vi "Data_PSD( Current Signal).vi"() -> ()   [LabVIEW 2020]
doc: "Use this template to build a producer/consumer design pattern. Use this template when you need to execute a process, such as data analysis, when a data source, such as a triggered acquisition, produces data at an uneven rate and you need to execute the process when the data becomes available."
uses:
  <vilib>/Utility/error.llb/DialogType.ctl
  <vilib>/measure/maspectr.llb/Power Spectrum and PSD Export Mode.ctl
  <vilib>/Analysis/4window.llb/windowTd.ctl
  <vilib>/DAQmx/read.llb/DAQmx Read (Analog Wfm 1Chan NSamp).vi
  <vilib>/DAQmx/create/channels.llb/DAQmx Create Channel (AI-Voltage-Basic).vi
  <vilib>/DAQmx/configure/timing.llb/DAQmx Timing (Sample Clock).vi
  <vilib>/DAQmx/miscellaneous.llb/DAQmx Fill In Error Info.vi
  <vilib>/measure/maspectr.llb/FFT Power Spectrum and PSD for 1 Chan.vi
  <vilib>/Analysis/0measdsp.llb/Scaled Time Domain Window (DBL).vi
  <vilib>/Analysis/NI_AALPro.lvlib
  <vilib>/measure/NI_MAPro.lvlib
panel:
  out "size(s)":i32
  out "Signal 2":waveform(dbl)(graph)
  in  "stop":bool
  out "Numeric":i32
  out "Signal":waveform(dbl)(graph)
  out "Max Amplitude":dbl
  out "PSD of Signal":cluster{"f0":dbl, "df":dbl, "S(f)":dbl[]}(graph)
  out "Frequency Peak":dbl format="%0.4f"
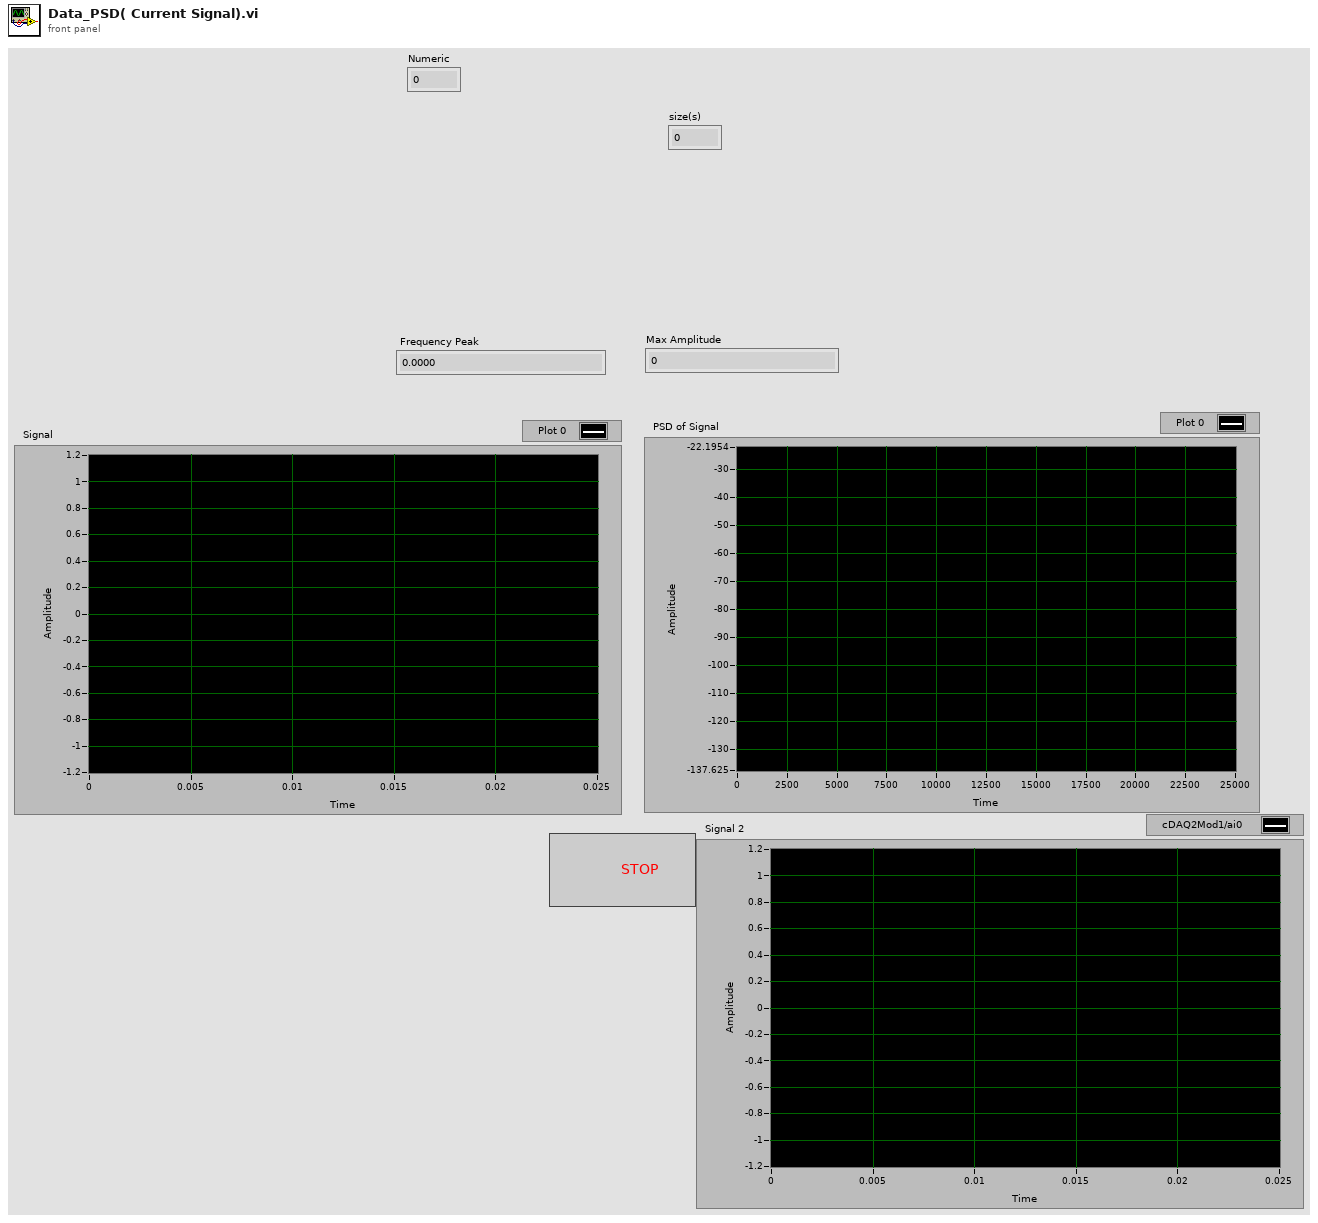
[diagram p1: front panel]
types:
  T1 = typedef "DialogType.ctl" = u16
  T2 = typedef "NI_AALPro.lvlib/windowTd.ctl" = u32
  T3 = typedef "NI_MAPro.lvlib/Power Spectrum and PSD Export Mode.ctl" = u16
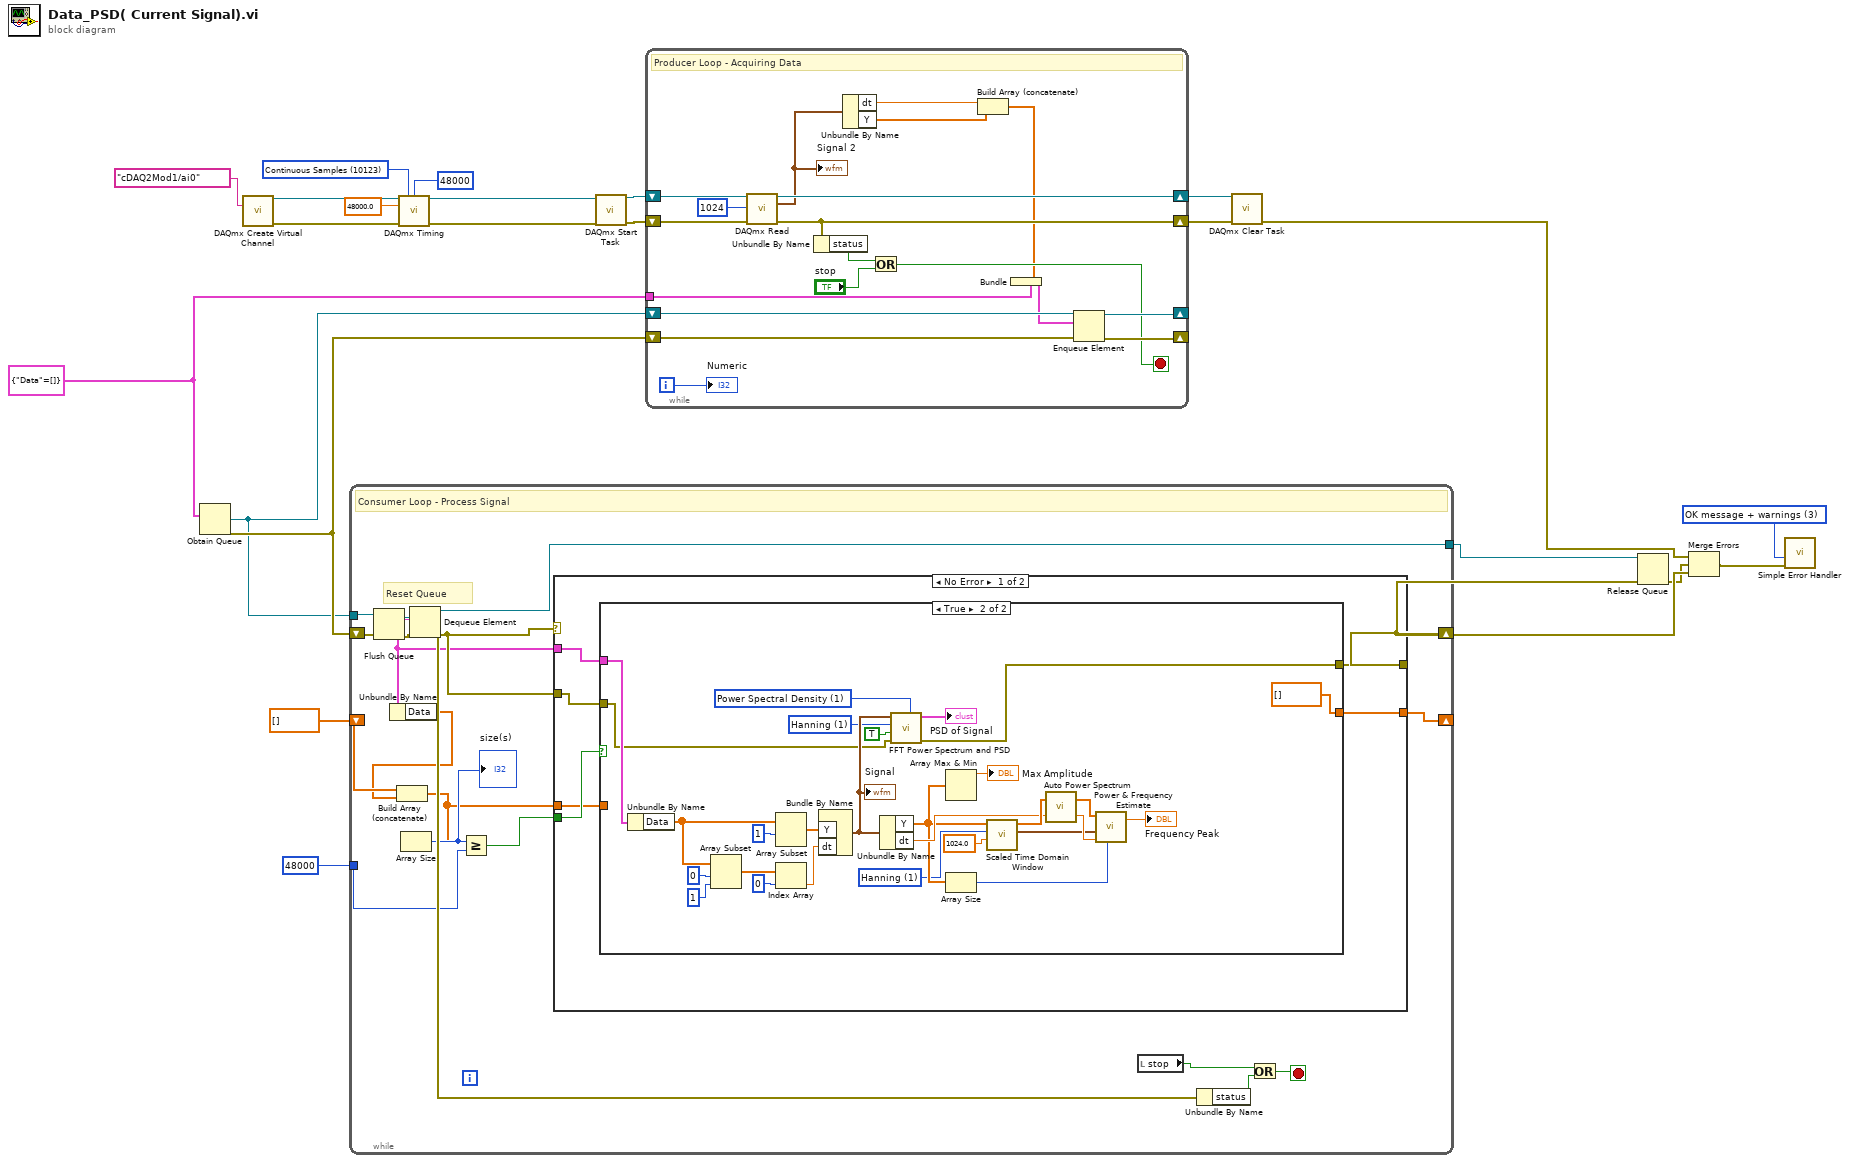
[diagram p0: block diagram]
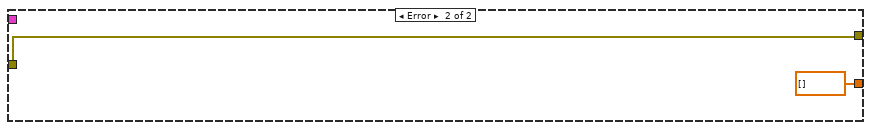
[diagram p3: hidden frame]
diagram:
  w3 = cluster{"Data":dbl[]} {"Data"=[]}
  w15 = 10123 items=["Finite Samples"=10178, "Continuous Samples"=10123, "Hardware Timed Single Point"=12522] ("sample mode")
  w23 = T1 3 items=["no dialog", "OK message", "continue or stop message", "OK message + warnings", "continue/stop + warnings"] ("type of dialog (OK msg:1)")
  n1 = Obtain Queue(element data type=w3) -> (queue out=w5:refnum<queue>, error out=w6:errorcluster)  [unwired: 3 in, 2 out]
  n2 = call-poly <vilib>:"DAQmx Create Virtual Channel.vi"("physical channels"=tag "cDAQ2Mod1/ai0") -> ("task out"=w17:refnum<k21>, "error out"=w16:errorcluster)  [unwired: 13 in]
  n3 = while {
    tunnel: w5 -> [w38]
    shift-right: [w41] -> w20
    shift-left: w6 -> [w36]
    tunnel: [w34] -> w21
    tunnel: 48000 -> [w29]
    shift-right: [w25] -> _
    shift-left: dbl[] [] -> [w30]
    stop <- w39 stop-if-true
    # "Reset Queue"
    # "Consumer Loop - Process Signal"
    n4 = Flush Queue(queue=w38, error in (no error)=w36) -> (queue out=w37:refnum<queue>, error out=w35:errorcluster)  [unwired: 1 out]
    n5 = Dequeue Element(queue=w37, error in (no error)=w35) -> (queue out=w34:refnum<queue>, element=w31:cluster{"Data":dbl[]}, error out=w33:errorcluster)  [unwired: 2 out]
    n6 = Unbundle By Name(w31) -> ("Data"=w26:dbl[])
    n7 = Build Array (concatenate)(w30, w26) -> (w24:dbl[])
    n8 = Array Size(array=w24) -> (size(s)=w28:i32)
    "size(s)" <- w28
    n9 = Greater Or Equal?(x=w28, y=w29) -> (x >= y?=w27:bool)
    n10 = case shown="No Error" w33 {
      tunnel: w31 -> [w47 _]
      tunnel: [w42 w79] -> w41
      tunnel: w33 -> [w43 w79]
      tunnel: w27 -> [w46 _]
      tunnel: [w45 dbl[] []] -> w25
      tunnel: w24 -> [w44 _]
      frame No Error {
        n11 = case shown="True" w46 {
          tunnel: w47 -> [_ w55]
          tunnel: [w49 dbl[] []] -> w45
          tunnel: w44 -> [w49 _]
          tunnel: w43 -> [w48 w51]
          tunnel: [w48 w50] -> w42
          frame False {
          }
          frame True {
            w56 = T2 1 items=["Rectangle"=0, "Hanning"=1, "Hamming"=2, "Blackman-Harris"=3, "Exact Blackman"=4, "Blackman"=5, "Flat Top"=6, "4 Term B-Harris "=7, "7 Term B-Harris"=8, "Low Sidelobe"=9, "Blackman Nuttall"=11, "Triangle"=30, "Bartlett-Hanning"=31, "Bohman"=32, "Parzen"=33, "Welch"=34, "Kaiser"=60, "Dolph-Chebyshev"=61, "Gaussian"=62] ("window")
            w57 = T2 1 items=["Rectangle"=0, "Hanning"=1, "Hamming"=2, "Blackman-Harris"=3, "Exact Blackman"=4, "Blackman"=5, "Flat Top"=6, "4 Term B-Harris "=7, "7 Term B-Harris"=8, "Low Sidelobe"=9, "Blackman Nuttall"=11, "Triangle"=30, "Bartlett-Hanning"=31, "Bohman"=32, "Parzen"=33, "Welch"=34, "Kaiser"=60, "Dolph-Chebyshev"=61, "Gaussian"=62] ("window")
            w72 = T3 1 items=["Power Spectrum", "Power Spectral Density"] ("export mode")
            n12 = Unbundle By Name(w55) -> ("Data"=w54:dbl[])
            n13 = Array Subset(array=w54, index=0, length=1) -> (w68:dbl[])
            n14 = Array Subset(array=w54, index=1) -> (w69:dbl[])  [unwired: 1 in]
            n15 = Index Array(array=w68, index=0) -> (element=w66:dbl)
            n16 = Bundle By Name("Y"=w69, "dt"=w66) -> (w61:waveform(dbl))  [unwired: 1 in]
            "Signal" <- w61
            n17 = Unbundle By Name(w61) -> ("Y"=w60:dbl[], "dt"=w71:dbl)
            n18 = call-poly <vilib>:"FFT Power Spectrum and PSD.vi"("export mode"=w72, "error in (no error)"=w51, "dB On (F)"=TRUE, "window"=w56, "time signal"=w61) -> ("error out"=w50:errorcluster, "Power Spectrum / PSD"=→"PSD of Signal":cluster{"f0":dbl, "df":dbl, "magnitude":dbl[]})  [unwired: 3 in, 2 out]
            n19 = Array Max & Min(array=w60) -> (max value=→"Max Amplitude":dbl)  [unwired: 3 out]
            n20 = Array Size(array=w60) -> (size(s)=w59:i32)
            n21 = call-poly <vilib>:"Scaled Time Domain Window.vi"("window parameter"=1024.0, "window"=w57, "X"=w60) -> ("window properties"=w58:cluster{"eq noise BW":dbl, "coherent gain":dbl}, "Windowed X"=w75:dbl[])  [unwired: 7 out]
            n22 = call <vilib>:"Auto Power Spectrum.vi"("dt"=w71, "Signal (V)"=w75) -> ("df"=w76:dbl, "Power Spectrum (V^2 rms)"=w63:dbl[])
            n23 = call <vilib>:"Power & Frequency Estimate.vi"("span"=w59, "df"=w76, "window constants"=w58, "Power Spectrum (V^2 rms)"=w63) -> ("est frequency peak"=→"Frequency Peak":dbl)  [unwired: 1 in, 2 out]
          }
        }
      }
      frame Error {
      }
    }
    n24 = local read "stop"() -> (w32:bool)
    n25 = Unbundle By Name(w33) -> ("status"=w40:bool)
    n26 = Or(x=w32, y=w40) -> (x .or. y?=w39:bool)
  }
  n27 = call-poly <vilib>:"DAQmx Timing.vi"("task/channels in"=w17, "sample mode"=w15, "samples per channel"=48000, "rate"=48000.0, "error in"=w16) -> ("task out"=w14:refnum<k21>, "error out"=w13:errorcluster)  [unwired: 9 in]
  n28 = call <vilib>:"DAQmx Start Task.vi"("task/channels in"=w14, "error in"=w13) -> ("task out"=w12:refnum<k21>, "error out"=w11:errorcluster)  [unwired: 12 in]
  n29 = while {
    shift-right: [w95] -> _
    shift-left: w6 -> [w96]
    shift-right: [w97] -> _
    shift-left: w5 -> [w98]
    shift-right: [w89] -> w9
    shift-left: w12 -> [w91]
    shift-right: [w88] -> w8
    shift-left: w11 -> [w90]
    tunnel: w3 -> [w84]
    i -> [w81]
    stop <- w92 stop-if-true
    # "Producer Loop - Acquiring Data"
    n30 = call-poly <vilib>:"DAQmx Read.vi"("task/channels in"=w91, "number of samples per channel"=1024, "error in"=w90) -> ("task out"=w89:refnum<k21>, "data"=w85:waveform(dbl), "error out"=w88:errorcluster)  [unwired: 10 in]
    "Signal 2" <- w85
    n31 = Unbundle By Name(w88) -> ("status"=w94:bool)
    n32 = Unbundle By Name(w85) -> ("dt"=w87:dbl, "Y"=w86:dbl[])
    n33 = Or(x=w94, y="stop") -> (x .or. y?=w92:bool)
    n34 = Build Array (concatenate)(w87, w86) -> (w83:dbl[])
    n35 = Bundle(cluster=w84, "Data"=w83) -> (w82:cluster{"Data":dbl[]})
    n36 = Enqueue Element(queue=w98, element=w82, error in (no error)=w96) -> (queue out=w97:refnum<queue>, error out=w95:errorcluster)  [unwired: 2 out]
    "Numeric" <- w81
  }
  n37 = call <vilib>:"DAQmx Clear Task.vi"("task in"=w9, "error in"=w8) -> ("error out"=w7:errorcluster)  [unwired: 13 out]
  n38 = Release Queue(queue=w21, error in (no error)=w20) -> (error out=w19:errorcluster)  [unwired: 1 in, 2 out]
  n39 = Merge Errors(w7, w19, w20) -> (w22:errorcluster)
  n40 = call <vilib>:"Simple Error Handler.vi"("type of dialog (OK msg:1)"=w23, "error in (no error)"=w22) -> ()  [unwired: 8 out]
